vi "Encoder_Count_To_Degrees.vi"(10 "Counts per Rev":dbl, 11 "Sensor Position":dbl) -> (3 "Degrees":dbl)   [LabVIEW 2020]
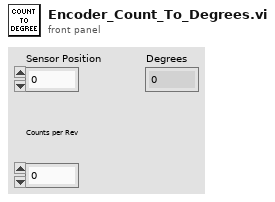
[diagram p1: front panel]
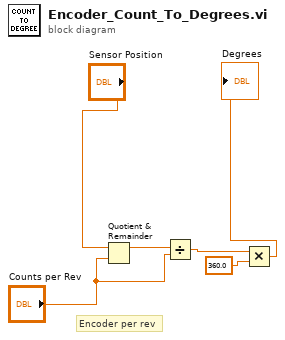
[diagram p0: block diagram]
diagram:
  # "Encoder per rev"
  n1 = Quotient & Remainder(x="Sensor Position", y="Counts per Rev") -> (x-y*floor(x/y)=w2:dbl)  [unwired: 1 out]
  n2 = Divide(x=w2, y="Counts per Rev") -> (x/y=w1:dbl)
  n3 = Multiply(x=w1, y=360.0) -> (x*y=→"Degrees":dbl)
